vi "Table Verify Cells.vi"(8 "error in (no error)":errorcluster, 9 "Table Datas 2D IN":string[][](array[string]), 10 "Title 1D IN":string[](array[string]), 11 "PdfP Table":refnum<k24>) -> (0 "error out":errorcluster, 1 "Table Datas 2D OUT":string[][](array[string]), 2 "Title 1D OUT":string[](array[string]), 3 "PdfP Table duplicate":refnum<k24>, 4 "ms":u32)   [LabVIEW 2013]
doc: "Version 1.0\nDeveloped by Jean-Marc Simard\nCopyright © 2010, Exaprom Inc.\nAll rights reserved.\nLicense: BSD\n\nWith iTextSharp 4.1.6 (http://itextsharp.sourceforge.net)\nunder Mozilla Public License Version 1.1\n(http://www.mozilla.org/MPL/MPL-1.1.html)"
uses:
  C:/Users/MaxCorp/Documents/GitHub/TopView/DLL/itextsharp.dll
  DLL/itextsharp.dll
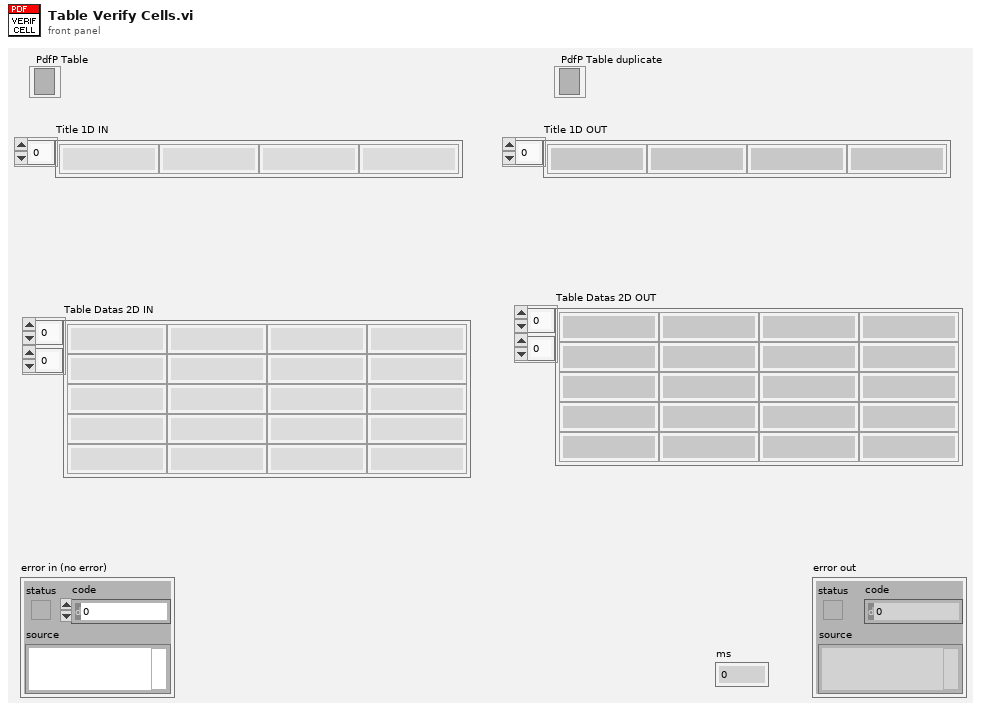
[diagram p1: front panel]
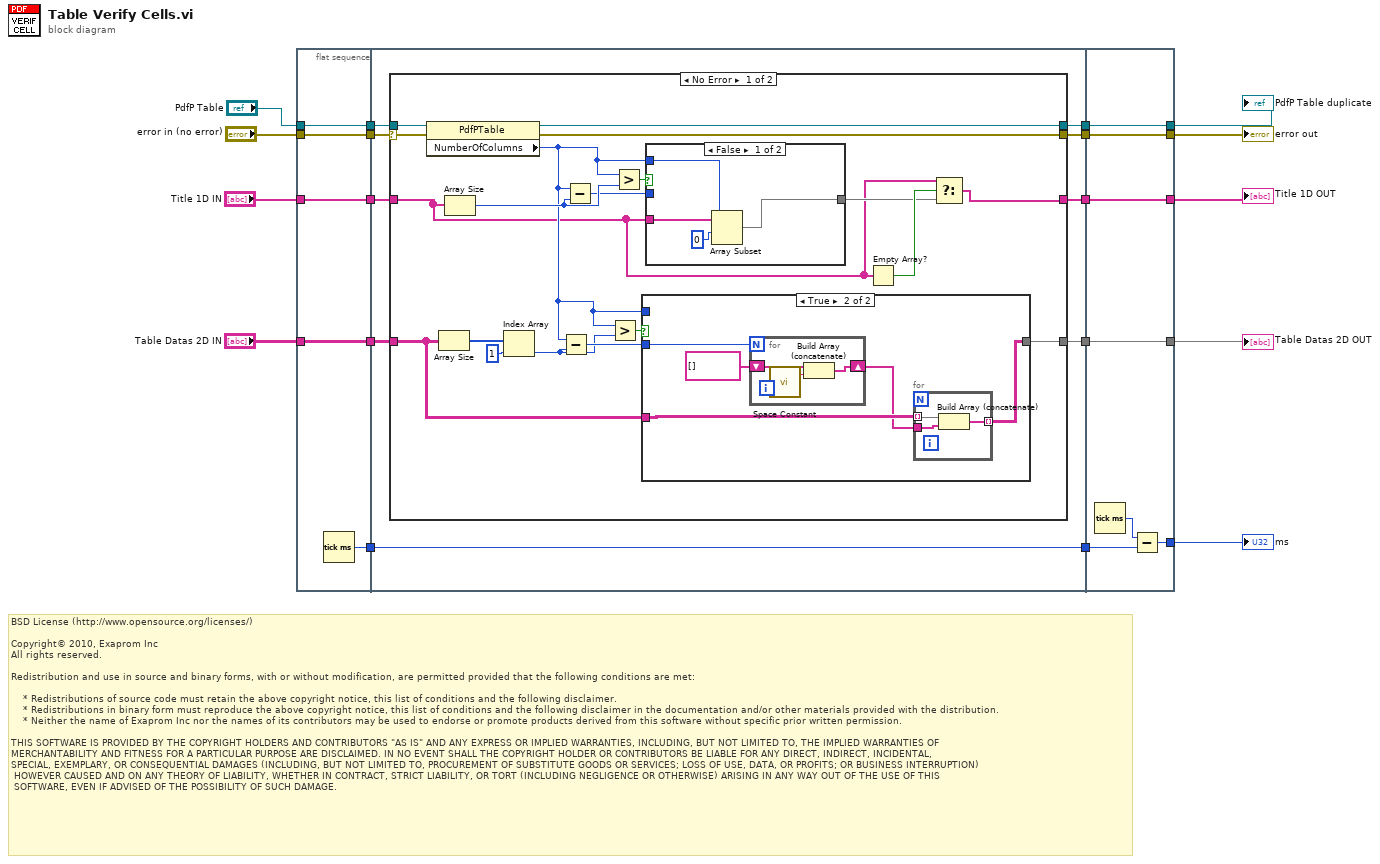
[diagram p0: block diagram]
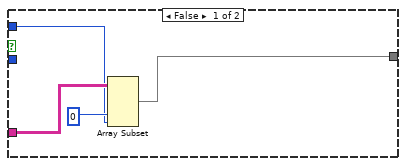
[diagram p2: hidden frame]
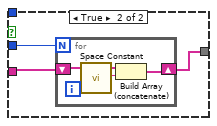
[diagram p3: hidden frame]
diagram:
  # "BSD License (http://www.opensource.org/licenses/)\n\nCopyright© 2010, Exaprom Inc\nAll rights reserved.\n\nRedistribution and use in source and binary forms, with or without modification, are permitted provided that the following conditions are met:\n\n    * Redistributions of source code must retain the above copyright notice, this list of conditions and the following disclaimer.\n    * Redistributions in binary form must reproduce the above copyright notice, this list of conditions and the following disclaimer in the documentation and/or other materials provided with the distribution.\n    * Neither the name of Exaprom Inc nor the names of its contributors may be used to endorse or promote products derived from this software without specific prior written permission.\n\nTHIS SOFTWARE IS PROVIDED BY THE COPYRIGHT HOLDERS AND CONTRIBUTORS \"AS IS\" AND ANY EXPRESS OR IMPLIED WARRANTIES, INCLUDING, BUT NOT LIMITED TO, THE IMPLIED WARRANTIES OF \nMERCHANTABILITY AND FITNESS FOR A PARTICULAR PURPOSE ARE DISCLAIMED. IN NO EVENT SHALL THE COPYRIGHT HOLDER OR CONTRIBUTORS BE LIABLE FOR ANY DIRECT, INDIRECT, INCIDENTAL,\nSPECIAL, EXEMPLARY, OR CONSEQUENTIAL DAMAGES (INCLUDING, BUT NOT LIMITED TO, PROCUREMENT OF SUBSTITUTE GOODS OR SERVICES; LOSS OF USE, DATA, OR PROFITS; OR BUSINESS INTERRUPTION)\n HOWEVER CAUSED AND ON ANY THEORY OF LIABILITY, WHETHER IN CONTRACT, STRICT LIABILITY, OR TORT (INCLUDING NEGLIGENCE OR OTHERWISE) ARISING IN ANY WAY OUT OF THE USE OF THIS\n SOFTWARE, EVEN IF ADVISED OF THE POSSIBILITY OF SUCH DAMAGE."
  n1 = flat-sequence {
    tunnel: "Table Datas 2D IN" -> [w21]
    tunnel: "Title 1D IN" -> [w22]
    tunnel: "PdfP Table" -> [w23]
    tunnel: "error in (no error)" -> [w24]
    tunnel: [w24] -> w11
    tunnel: [w23] -> w10
    tunnel: [w22] -> w9
    tunnel: [w21] -> w8
    tunnel: [w20] -> w3
    tunnel: w11 -> [w32]
    tunnel: w10 -> [w31]
    tunnel: w9 -> [w30]
    tunnel: w8 -> [w29]
    tunnel: [w33] -> w7
    tunnel: [w28] -> w6
    tunnel: [w27] -> w5
    tunnel: [w26] -> w4
    tunnel: w3 -> [w25]
    tunnel: [w25] -> w2
    tunnel: [w85] -> w12
    tunnel: [w86] -> w13
    tunnel: [w87] -> w14
    tunnel: [w88] -> w19
    tunnel: w7 -> [w88]
    tunnel: w6 -> [w87]
    tunnel: w5 -> [w86]
    tunnel: w4 -> [w85]
    tunnel: w2 -> [w83]
    tunnel: [w82] -> w1
    frame #0 {
      n2 = Tick Count (ms)() -> (millisecond timer value=w20:u32)
    }
    frame #1 {
      n3 = case shown="No Error" w32 {
        selector: w32 -> [w51 w81]
        tunnel: [w48 w81] -> w33
        tunnel: w31 -> [w52 w78]
        tunnel: w30 -> [w34 w80]
        tunnel: w29 -> [w41 w79]
        tunnel: [w35 w80] -> w27
        tunnel: [w40 w79] -> w28
        tunnel: [w38 w78] -> w26
        frame No Error {
          n4 = property class="PdfPTable"(reference=w52, error in=w51) -> (reference out=w38:refnum<k24>, error out=w48:errorcluster, "NumberOfColumns"=w39:i32)
          n5 = Array Size(array=w41) -> (size(s)=w50:i32[])
          n6 = Array Size(array=w34) -> (size(s)=w46:i32)
          n7 = Index Array(array=w50, index=1) -> (element=w42:i32)
          n8 = Subtract(x=w39, y=w42) -> (x-y=w44:i32)
          n9 = Subtract(x=w39, y=w46) -> (x-y=w45:i32)
          n10 = Greater?(x=w39, y=w42) -> (0:w43:bool)
          n11 = Greater?(x=w39, y=w46) -> (0:w47:bool)
          n12 = case shown="True" w43 {
            tunnel: w41 -> [w56 w59]
            tunnel: w39 -> [w53 _]
            tunnel: w44 -> [_ w61]
            tunnel: [w55 w58] -> w40
            frame False {
              n13 = Array Subset(array=w56, index (col)=0 ("index"), length (col)=w53) -> (w55:string[][])  [unwired: 2 in]
            }
            frame True {
              n14 = for {
                N: w61 -> [_]
                shift-right: [w67] -> w57
                shift-left: string[] [] -> [w66]
                n15 = call <vilib>:"Space Constant.vi"() -> ("String"=w65:string)
                n16 = Build Array (concatenate)(w66, w65) -> (w67:string[])
              }
              n17 = for {
                tunnel: w59 -> [w63] mode=indexing
                tunnel: [w64] -> w58 mode=indexing
                tunnel: w57 -> [w62]
                n18 = Build Array (concatenate)(w63, w62) -> (w64:string[])
              }
            }
          }
          n19 = case shown="False" w47 {
            tunnel: w34 -> [w71 w73]
            tunnel: w39 -> [w69 _]
            tunnel: w45 -> [_ w74]
            tunnel: [w70 w72] -> w36
            frame False {
              n20 = Array Subset(array=w71, index=0, length=w69) -> (w70:string[])
            }
            frame True {
              n21 = for {
                N: w74 -> [_]
                shift-right: [w76] -> w72
                shift-left: w73 -> [w77]
                n22 = call <vilib>:"Space Constant.vi"() -> ("String"=w75:string)
                n23 = Build Array (concatenate)(w77, w75) -> (w76:string[])
              }
            }
          }
          n24 = Empty Array?(array=w34) -> (empty?=w37:bool)
          n25 = Select(t=w34, s=w37, f=w36) -> (s? t:f=w35:string[])
        }
        frame Error {
        }
      }
    }
    frame #2 {
      n26 = Tick Count (ms)() -> (millisecond timer value=w84:u32)
      n27 = Subtract(x=w84, y=w83) -> (x-y=w82:u32)
    }
  }
  "error out" <- w19
  "Title 1D OUT" <- w13
  "Table Datas 2D OUT" <- w14
  "PdfP Table duplicate" <- w12
  "ms" <- w1
